vi "Constructor.vi"(8 "error in":errorcluster, 10 "Comparison":bool, 11 "Name":string) -> (0 "error out":errorcluster, 3 "BooleanMeasureLimit":refnum<class "BooleanMeasureLimit.lvclass">)   [LabVIEW 2021, in "ProligentXMLGenerator.lvlib" / "BooleanMeasureLimit.lvclass"]
uses:
  BooleanMeasureLimit.lvclass
  BooleanMeasureLimit.lvclass/BooleanMeasureLimit.ctl
  MeasureLimit/MeasureLimit.lvclass
  Data.ctl
  Base/Boolean/Boolean.lvclass
  C:/Projects/proligent-xml-generator-labview/src/ProligentXMLGenerator/Measure/MeasureLimit/MeasureLimit.lvclass
  C:/Projects/proligent-xml-generator-labview/src/ProligentXMLGenerator/Measure/BooleanMeasureLimit/BooleanMeasureLimit.lvclass
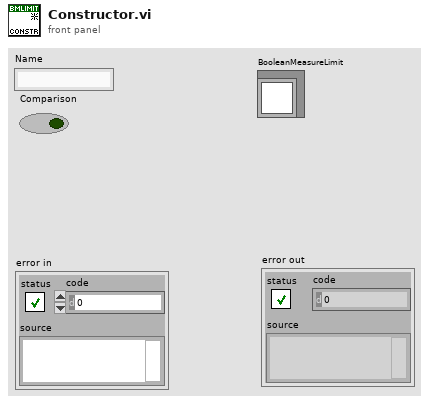
[diagram p1: front panel]
types:
  T1 = typedef "ProligentXMLGenerator.lvlib/BooleanMeasureLimit.lvclass/Data.ctl" = cluster{"Comparison":refnum<class "Boolean.lvclass">}
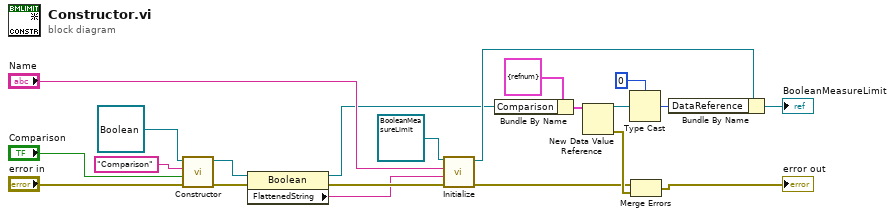
[diagram p0: block diagram]
diagram:
  n1 = call-dynamic "Constructor.vi"("error in"="error in", "Value"="Comparison", "Name"="Comparison", "Boolean in"=refnum<class "Boolean.lvclass"> refnum ("ProligentResultProcessor:Boolean")) -> ("error out"=w6:errorcluster, "Boolean out"=w3:refnum<class "Boolean.lvclass">)  [unwired: 6 in]
  n2 = property on="Property Node" class="Boolean"(reference=w3, error in=w6) -> (reference out=w2:refnum<class "Boolean.lvclass">, error out=w4:errorcluster, "FlattenedString"=w1:string)
  n3 = call "Initialize.vi"("error in"=w4, "LimitExpression"=w1, "Name"="Name", "MeasureLimit in"=refnum<class "BooleanMeasureLimit.lvclass"> refnum ("ProligentResultProcessor:BooleanMeasureLimit")) -> ("error out"=w13:errorcluster, "MeasureLimit out"=w12:refnum<class "BooleanMeasureLimit.lvclass">)  [unwired: 6 in]
  n4 = Bundle By Name(cluster=T1 {"Comparison"=refnum} ("Data"), "Comparison"=w2) -> (w17:T1)
  n5 = New Data Value Reference(data value=w17) -> (data value reference=w18:refnum<data-value>, error out=w21:errorcluster)  [unwired: 1 in]
  n6 = Type Cast(type=u64 0, x=w18) -> (*(type *) &x=w20:u64)
  n7 = Merge Errors(w13, w21) -> (→"error out":errorcluster)
  n8 = Bundle By Name(cluster=w12, "DataReference"=w20) -> (→"BooleanMeasureLimit":refnum<class "BooleanMeasureLimit.lvclass">)
